vi "Check.vi"(11 "DataIn":T1) -> (0 "True = Empatou":bool, 3 "True = Ganhou":bool)   [LabVIEW 2017]
doc: "SubVI criado para checar se houve vitória ou empate através de comparação das posiçõs da matriz do tabuleiro."
uses:
  controls/DataIn.ctl
  controls/Tabuleiro.ctl
  controls/GameOption.ctl
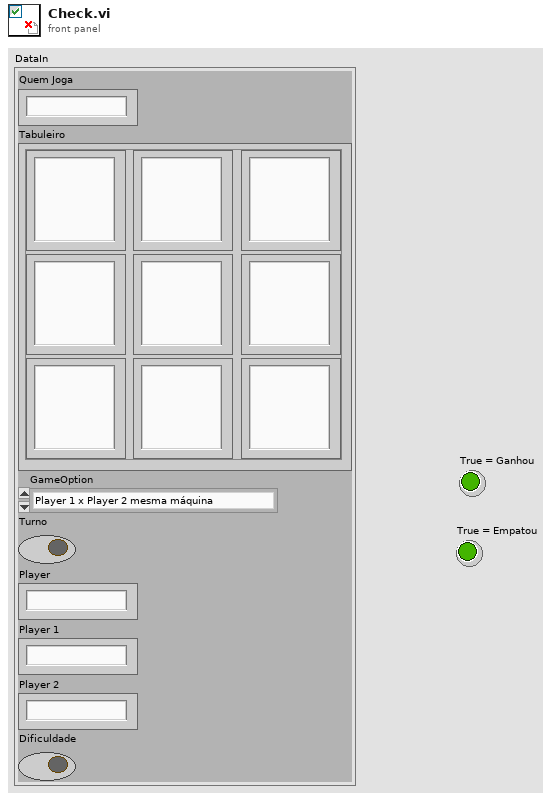
[diagram p1: front panel]
types:
  T1 = typedef "DataIn.ctl" = cluster{"Quem Joga":string, "Tabuleiro":T2, "GameOption":T3, "Turno":bool, "Player":string, "Player 1":string, "Player 2":string, "Dificuldade":bool}
  T2 = typedef "Tabuleiro.ctl" = cluster{"(0,0)":string, "(1,0)":string, "(0,1)":string, "(1,1)":string, "(2,0)":string, "(1,2)":string, "(2,2)":string, "(0,2)":string, "(2,1) ":string}
  T3 = typedef "GameOption.ctl" = enum16{"Player 1 x Player 2 mesma máquina", "Player 1 x Player 2 pela rede", "Player 1 x Computador", "Wait for Event", "Initialize"}
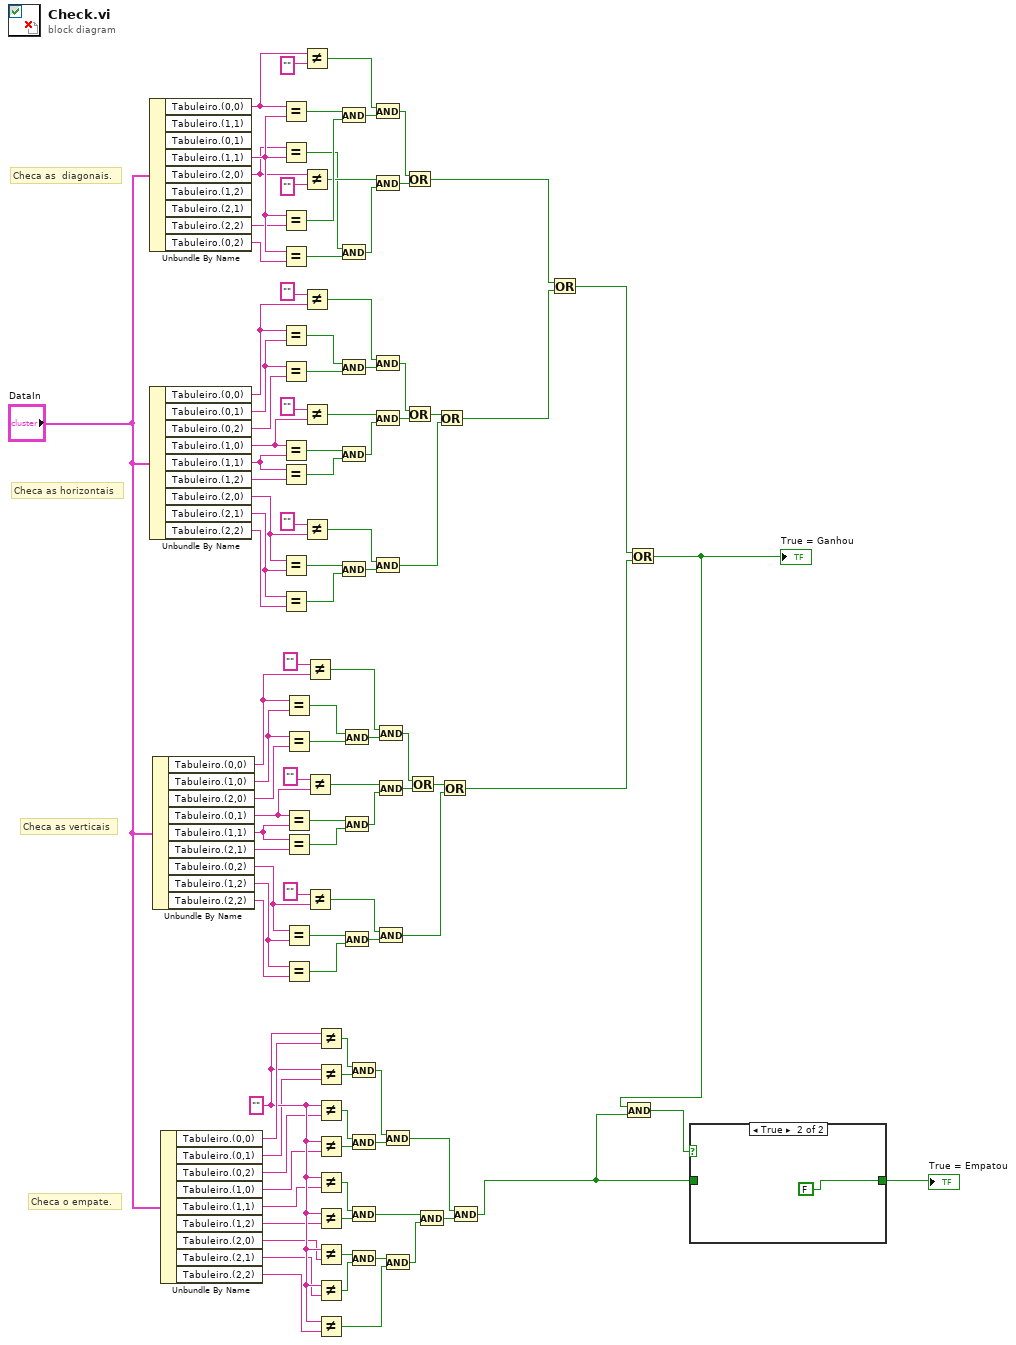
[diagram p0: block diagram]
diagram:
  w31 = "" ("y")
  # "Checa as verticais"
  # "Checa as horizontais"
  # "Checa o empate."
  # "Checa as  diagonais."
  n1 = Unbundle By Name("DataIn") -> ("Tabuleiro.(0,0)"=w104:string, "Tabuleiro.(1,1)"=w107:string, "Tabuleiro.(2,0)"=w106:string, "Tabuleiro.(2,2)"=w105:string, "Tabuleiro.(0,2)"=w108:string)  [unwired: 4 out]
  n2 = Unbundle By Name("DataIn") -> ("Tabuleiro.(0,0)"=w90:string, "Tabuleiro.(0,1)"=w89:string, "Tabuleiro.(0,2)"=w88:string, "Tabuleiro.(1,0)"=w82:string, "Tabuleiro.(1,1)"=w81:string, "Tabuleiro.(1,2)"=w80:string, "Tabuleiro.(2,0)"=w74:string, "Tabuleiro.(2,1)"=w72:string, "Tabuleiro.(2,2)"=w73:string)
  n3 = Unbundle By Name("DataIn") -> ("Tabuleiro.(0,0)"=w62:string, "Tabuleiro.(1,0)"=w61:string, "Tabuleiro.(2,0)"=w60:string, "Tabuleiro.(0,1)"=w54:string, "Tabuleiro.(1,1)"=w53:string, "Tabuleiro.(2,1)"=w52:string, "Tabuleiro.(0,2)"=w46:string, "Tabuleiro.(1,2)"=w44:string, "Tabuleiro.(2,2)"=w45:string)
  n4 = Unbundle By Name("DataIn") -> ("Tabuleiro.(0,0)"=w32:string, "Tabuleiro.(0,1)"=w30:string, "Tabuleiro.(0,2)"=w29:string, "Tabuleiro.(1,0)"=w28:string, "Tabuleiro.(1,1)"=w27:string, "Tabuleiro.(1,2)"=w26:string, "Tabuleiro.(2,0)"=w25:string, "Tabuleiro.(2,1)"=w24:string, "Tabuleiro.(2,2)"=w1:string)
  n5 = Equal?(x=w104, y=w107) -> (x = y?=w99:bool)
  n6 = Equal?(x=w106, y=w107) -> (x = y?=w95:bool)
  n7 = Equal?(x=w107, y=w105) -> (x = y?=w98:bool)
  n8 = Equal?(x=w107, y=w108) -> (x = y?=w94:bool)
  n9 = Equal?(x=w90, y=w89) -> (x = y?=w87:bool)
  n10 = Equal?(x=w89, y=w88) -> (x = y?=w86:bool)
  n11 = Equal?(x=w82, y=w81) -> (x = y?=w79:bool)
  n12 = Equal?(x=w81, y=w80) -> (x = y?=w78:bool)
  n13 = Equal?(x=w74, y=w72) -> (x = y?=w71:bool)
  n14 = Equal?(x=w72, y=w73) -> (x = y?=w70:bool)
  n15 = Equal?(x=w62, y=w61) -> (x = y?=w59:bool)
  n16 = Equal?(x=w61, y=w60) -> (x = y?=w58:bool)
  n17 = Equal?(x=w54, y=w53) -> (x = y?=w51:bool)
  n18 = Equal?(x=w53, y=w52) -> (x = y?=w50:bool)
  n19 = Equal?(x=w46, y=w44) -> (x = y?=w43:bool)
  n20 = Equal?(x=w44, y=w45) -> (x = y?=w42:bool)
  n21 = Not Equal?(x=w104, y="") -> (x != y?=w101:bool)
  n22 = Not Equal?(x=w106, y="") -> (x != y?=w96:bool)
  n23 = Not Equal?(x="" ("y"), y=w90) -> (x != y?=w85:bool)
  n24 = Not Equal?(x="" ("y"), y=w82) -> (x != y?=w76:bool)
  n25 = Not Equal?(x="" ("y"), y=w74) -> (x != y?=w68:bool)
  n26 = Not Equal?(x="" ("y"), y=w62) -> (x != y?=w57:bool)
  n27 = Not Equal?(x="" ("y"), y=w54) -> (x != y?=w48:bool)
  n28 = Not Equal?(x="" ("y"), y=w46) -> (x != y?=w40:bool)
  n29 = Not Equal?(x=w31, y=w32) -> (x != y?=w23:bool)
  n30 = Not Equal?(x=w31, y=w30) -> (x != y?=w22:bool)
  n31 = Not Equal?(x=w31, y=w29) -> (x != y?=w21:bool)
  n32 = Not Equal?(x=w31, y=w28) -> (x != y?=w20:bool)
  n33 = Not Equal?(x=w31, y=w27) -> (x != y?=w19:bool)
  n34 = Not Equal?(x=w31, y=w26) -> (x != y?=w18:bool)
  n35 = Not Equal?(x=w31, y=w25) -> (x != y?=w17:bool)
  n36 = Not Equal?(x=w31, y=w24) -> (x != y?=w16:bool)
  n37 = Not Equal?(x=w31, y=w1) -> (x != y?=w15:bool)
  n38 = And(x=w99, y=w98) -> (x .and. y?=w100:bool)
  n39 = And(x=w95, y=w94) -> (x .and. y?=w97:bool)
  n40 = And(x=w87, y=w86) -> (x .and. y?=w84:bool)
  n41 = And(x=w79, y=w78) -> (x .and. y?=w77:bool)
  n42 = And(x=w71, y=w70) -> (x .and. y?=w69:bool)
  n43 = And(x=w59, y=w58) -> (x .and. y?=w56:bool)
  n44 = And(x=w51, y=w50) -> (x .and. y?=w49:bool)
  n45 = And(x=w43, y=w42) -> (x .and. y?=w41:bool)
  n46 = And(x=w23, y=w22) -> (x .and. y?=w11:bool)
  n47 = And(x=w21, y=w20) -> (x .and. y?=w10:bool)
  n48 = And(x=w19, y=w18) -> (x .and. y?=w12:bool)
  n49 = And(x=w17, y=w16) -> (x .and. y?=w14:bool)
  n50 = And(x=w101, y=w100) -> (x .and. y?=w102:bool)
  n51 = And(x=w96, y=w97) -> (x .and. y?=w103:bool)
  n52 = And(x=w85, y=w84) -> (x .and. y?=w67:bool)
  n53 = And(x=w76, y=w77) -> (x .and. y?=w66:bool)
  n54 = And(x=w68, y=w69) -> (x .and. y?=w65:bool)
  n55 = And(x=w57, y=w56) -> (x .and. y?=w39:bool)
  n56 = And(x=w48, y=w49) -> (x .and. y?=w38:bool)
  n57 = And(x=w40, y=w41) -> (x .and. y?=w37:bool)
  n58 = And(x=w11, y=w10) -> (x .and. y?=w9:bool)
  n59 = And(x=w14, y=w15) -> (x .and. y?=w13:bool)
  n60 = Or(x=w102, y=w103) -> (x .or. y?=w35:bool)
  n61 = Or(x=w67, y=w66) -> (x .or. y?=w64:bool)
  n62 = Or(x=w39, y=w38) -> (x .or. y?=w36:bool)
  n63 = And(x=w12, y=w13) -> (x .and. y?=w8:bool)
  n64 = Or(x=w64, y=w65) -> (x .or. y?=w34:bool)
  n65 = Or(x=w36, y=w37) -> (x .or. y?=w7:bool)
  n66 = And(x=w9, y=w8) -> (x .and. y?=w6:bool)
  n67 = Or(x=w35, y=w34) -> (x .or. y?=w33:bool)
  n68 = Or(x=w33, y=w7) -> (x .or. y?=w3:bool)
  "True = Ganhou" <- w3
  n69 = And(x=w3, y=w6) -> (x .and. y?=w5:bool)
  n70 = case shown="True" w5 {
    tunnel: w6 -> [w109 _]
    tunnel: [w109 FALSE] -> w4
    frame False {
    }
    frame True {
    }
  }
  "True = Empatou" <- w4
